vi "Finish.vi"   [LabVIEW 2013]
doc: "This VI is called just before exiting. It is expected to close I/O refnum, save collected data, etc."
uses:
  <vilib>/Rock Robotics/WPI/RobotDrive/WPI_RobotDriveGetSetRefNum.vi
  <vilib>/Rock Robotics/WPI/Joystick/WPI_JoystickGetSetRefNum.vi
types:
  T1 = typedef "WPI_RelayDevRef.ctl" = cluster{"DevStatus":errorcluster, "Relay Channel":T2, "Digital Module":T3, "Relay Direction":T4}
  T2 = typedef "FPGA_DIORelayChannel.ctl" = enum8{"Relay 1", "Relay 2", "Relay 3", "Relay 4", "Relay 5", "Relay 6", "Relay 7", "Relay 8", "Invalid"}
  T3 = typedef "FPGA_TypedefDigitalModule.ctl" = enum16{"Digital Module 1", "Digital Module 2"}
  T4 = typedef "WPI_RelayDirection.ctl" = enum16{"Both directions", "Forward only", "Reverse only"}
  T5 = typedef "WPI_JoystickDevRef.ctl" = cluster{"Device":T6}
  T6 = typedef "WPI_JoystickDeviceEnum.ctl" = enum16{"USB 1", "USB 2", "USB 3", "USB 4", "Kinect 1", "Kinect 2"}
  T7 = typedef "WPI_RobotDriveDevRef.ctl" = cluster{"DevStatus":errorcluster, "Motors[]":T8[], "Square Inputs":bool, "Max Output":dbl, "Isochronous":bool}
  T8 = typedef "WPI_MotorControlDeviceRef.ctl" = cluster{"DeviceStatus":errorcluster, "Type":enum16{"PWM", "CAN"}, "PWM":cluster{"Digital Module":T3, "PWM Channel":T9, "DeadBand":T10}, "CAN":cluster{"Device Number":u8, "Control Mode":T11, "Semaphore":T12, "Max Vout":dbl}, "Invert":bool, "TransformRef":T13, "InvTransformRef":T13}
  T9 = typedef "FPGA_DIOPWMChannel.ctl" = enum8{"PWM 1", "PWM 2", "PWM 3", "PWM 4", "PWM 5", "PWM 6", "PWM 7", "PWM 8", "PWM 9", "PWM 10", "Invalid"}
  T10 = typedef "WPI_PWMDeadband.ctl" = cluster{"Name":string, "maxPositivePwm":i32, "minPositivePwm":i32, "centerPwm":i32, "maxNegativePwm":i32, "minNegativePwm":i32, "angularRange":u16}
  T11 = typedef "WPI_CANJaguar_ControlMode.ctl" = enum8{"Percent VBus", "Current", "Speed", "Position", "Voltage"}
  T12 = typedef "Semaphore RefNum" = refnum<k1>
  T13 = typedef "WPI_PWMTransform_ConPane.ctl" = refnum<vi>
  T14 = typedef "WPI_EncoderDevRef.ctl" = cluster{"DevStatus":errorcluster, "EncoderIndex":T15, "CounterIndex":T16, "DistancePerCount":dbl, "Decoding Type":T17}
  T15 = typedef "FPGA_EncoderIdx.ctl" = enum8{"Enc 0", "Enc 1", "Enc 2", "Enc 3", "Invalid"}
  T16 = typedef "FPGA_CounterCtrSystemIndex.ctl" = enum8{"Ctr 0", "Ctr 1", "Ctr 2", "Ctr 3", "Ctr 4", "Ctr 5", "Ctr 6", "Ctr 7", "Invalid"}
  T17 = typedef "WPI_EncoderType.ctl" = enum16{"1x", "2x", "4x"}
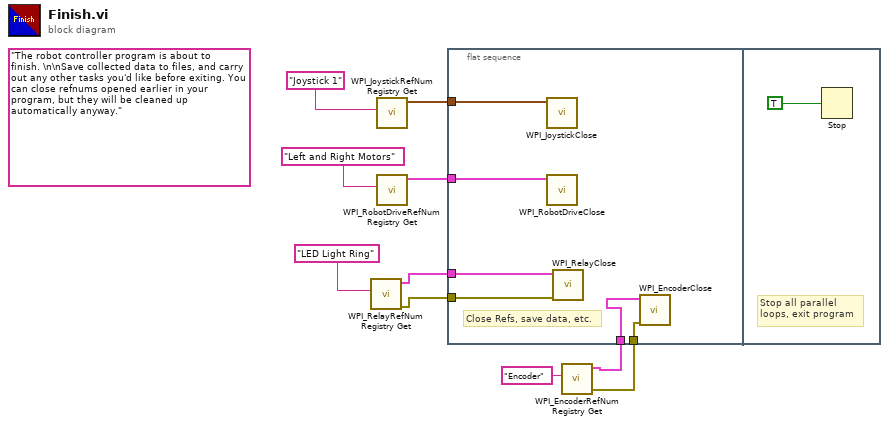
[diagram p0: block diagram]
diagram:
  (unwired) "The robot controller program is about to finish. \n\nSave collected data to files, and carry out any other tasks you'd like before exiting. You can close refnums opened earlier in your program, but they will be cleaned up automatically anyway."
  n1 = call <vilib>:"WPI_RelayRefNum Registry Get.vi"("refnum name"="LED Light Ring") -> ("error out"=w4:errorcluster, "RelayDevRef"=w5:T1)  [unwired: 9 in]
  n2 = call <vilib>:"WPI_JoystickRefNum Registry Get.vi"("refnum name"="Joystick 1") -> ("JoystickDevRef"=w7:T5)  [unwired: 1 in, 9 out]
  n3 = call <vilib>:"WPI_RobotDriveRefNum Registry Get.vi"("refnum name"="Left and Right Motors") -> ("RobotDriveDevRef"=w8:T7)  [unwired: 1 in, 9 out]
  n4 = flat-sequence {
    tunnel: w8 -> [w16]
    tunnel: w7 -> [w15]
    tunnel: w5 -> [w14]
    tunnel: w4 -> [w13]
    tunnel: w3 -> [w12]
    tunnel: w2 -> [w11]
    frame #0 {
      # "Close Refs, save data, etc."
      n5 = call <vilib>:"WPI_JoystickClose.vi"("JoystickDevRef"=w15) -> ()  [unwired: 11 out]
      n6 = call <vilib>:"WPI_RobotDriveClose.vi"("RobotDriveDevRef"=w16) -> ()  [unwired: 1 in, 10 out]
      n7 = call <vilib>:"WPI_RelayClose.vi"("error in (no error)"=w13, "RelayDevRef"=w14) -> ()  [unwired: 9 in, 1 out]
      n8 = call <vilib>:"WPI_EncoderClose.vi"("error in (no error)"=w11, "EncoderDevRef"=w12) -> ()  [unwired: 9 in, 1 out]
    }
    frame #1 {
      # "Stop all parallel\nloops, exit program"
      n9 = Stop(stop? (T)=TRUE ("Quit")) -> ()
    }
  }
  n10 = call <vilib>:"WPI_EncoderRefNum Registry Get.vi"("refnum name"="Encoder") -> ("error out"=w2:errorcluster, "EncoderDevRef"=w3:T14)  [unwired: 9 in]
